vi "3DexampleCode.vi"() -> ()   [LabVIEW 2010]
uses:
  <vilib>/picture/3D Picture Control/NI_3D Picture Control.lvlib
panel:
  out "3D Picture":refnum<vi>(3d-picture)
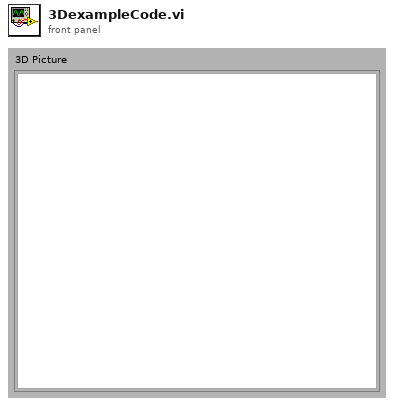
[diagram p1: front panel]
types:
  T1 = cluster{"Red":sgl, "Green":sgl, "Blue":sgl, "Alpha":sgl}
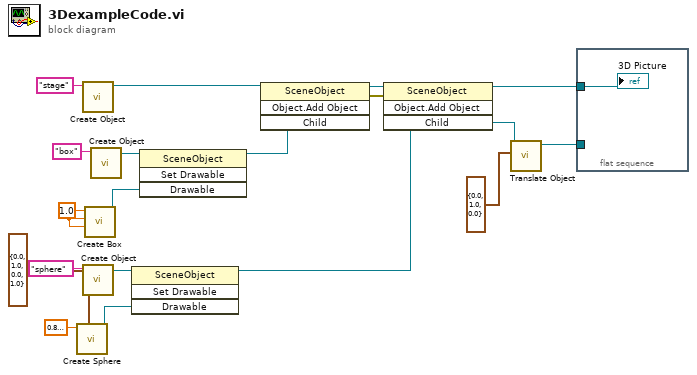
[diagram p0: block diagram]
diagram:
  w13 = sgl 1.0 ("Radius")
  n1 = call <vilib>:"Create Sphere.vi"("Color"=T1 {"Red"=0.0, "Green"=1.0, "Blue"=0.0, "Alpha"=1.0}, "Radius"=sgl 0.8) -> ("New Sphere Refnum"=w11:refnum<vi>)  [unwired: 8 in, 1 out]
  n2 = call <vilib>:"Create Object.vi"("Name"="stage") -> ("Scene:New Object"=w15:refnum<vi>)  [unwired: 1 in, 9 out]
  n3 = call <vilib>:"Create Object.vi"("Name"="sphere") -> ("Scene:New Object"=w10:refnum<vi>)  [unwired: 1 in, 9 out]
  n4 = call <vilib>:"Create Box.vi"("Length Z"=w13, "Length Y"=w13, "Length X"=w13) -> ("New Box Refnum"=w18:refnum<vi>)  [unwired: 7 in, 1 out]
  n5 = call <vilib>:"Create Object.vi"("Name"="box") -> ("Scene:New Object"=w19:refnum<vi>)  [unwired: 1 in, 9 out]
  n6 = invoke class="SceneObject" method="Set Drawable"(reference=w10, "Drawable"=w11) -> (reference out=w6:refnum<vi>)  [unwired: 2 in, 3 out]
  n7 = invoke class="SceneObject" method="Set Drawable"(reference=w19, "Drawable"=w18) -> (reference out=w14:refnum<vi>)  [unwired: 2 in, 3 out]
  n8 = invoke class="SceneObject" method="Object.Add Object"(reference=w15, "Child"=w14) -> (reference out=w7:refnum<vi>, error out=w8:errorcluster)  [unwired: 2 in, 2 out]
  n9 = invoke class="SceneObject" method="Object.Add Object"(reference=w7, error in=w8, "Child"=w6) -> (reference out=w5:refnum<vi>, "Child"=w3:refnum<vi>)  [unwired: 1 in, 2 out]
  n10 = call <vilib>:"Translate Object.vi"("Translation"=cluster{"X":sgl, "Y":sgl, "Z":sgl} {"X"=0.0, "Y"=1.0, "Z"=0.0}, "Scene.Object In"=w3) -> ("Scene.Object Out"=w1:refnum<vi>)  [unwired: 8 in, 1 out]
  n11 = flat-sequence {
    tunnel: w5 -> [w20]
    tunnel: w1 -> [_]
    frame #0 {
      "3D Picture" <- w20
    }
  }
